vi "go.vi"(10 "string":string="Hello World !", 11 "milliseconds to wait":u32) -> (2 "Numeric":i32)   [LabVIEW 2015]
panel:
  out "String":string
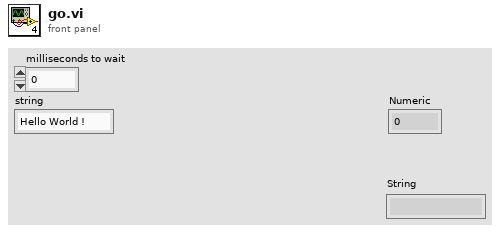
[diagram p1: front panel]
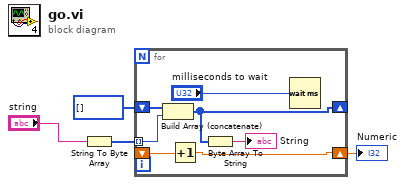
[diagram p0: block diagram]
diagram:
  n1 = String To Byte Array(string="string") -> (unsigned byte array=w3:u8[])
  n2 = for {
    tunnel: w3 -> [w10] mode=indexing
    shift-right: [w9] -> _
    shift-left: u8[] [] -> [w11]
    shift-right: [w5] -> w1
    shift-left: _ -> [w6]
    n3 = Build Array (concatenate)(w11, w10) -> (w9:u8[])
    n4 = Increment(x=w6) -> (x+1=w5:dbl)
    n5 = Byte Array To String(unsigned byte array=w9) -> (string=→"String":string)
    n6 = Wait (ms)(milliseconds to wait="milliseconds to wait") -> ()  [unwired: 1 out]
  }
  "Numeric" <- w1
